vi "Close Panel With Fade Out.vi"(8 "error in":errorcluster, 11 "Philips Dialog in":refnum<class "Flex UI Dialog.lvclass">) -> (0 "error out":errorcluster, 3 "Philips Dialog out":refnum<class "Flex UI Dialog.lvclass">)   [LabVIEW 2014, in "Flex UI Dialog.lvclass"]
doc: "If the dialog front panel was initially closed, close it. Otherwise do nothing."
uses:
  Flex UI Dialog.lvclass
  Flex UI Dialog.lvclass/Flex UI Dialog.ctl
  Flex UI (Parent)/Flex UI.lvclass/Flex UI.ctl
  <vilib>/LAVA/UI Tools/Fading/_Fade(I32)__lava_lib_ui_tools.vi
  Flex UI (Parent)/Flex UI.lvclass
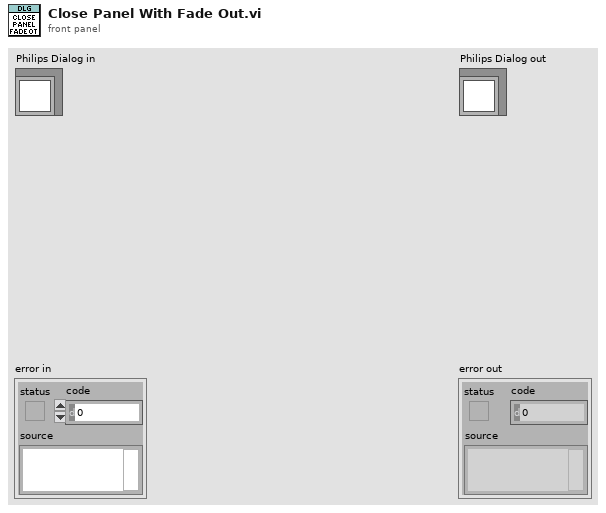
[diagram p1: front panel]
types:
  T1 = enum32{"invalid app kind", "Development System", "Run Time System", "Student Edition", "Embedded LabVIEW", "Evaluation", "Custom"}
  T2 = enum32{"Invalid", "Default", "Floating", "Floating/Auto-Hide", "Modal"}
  T3 = enum32{"Invalid", "Standard", "Closed", "Hidden", "Minimized", "Maximized"}
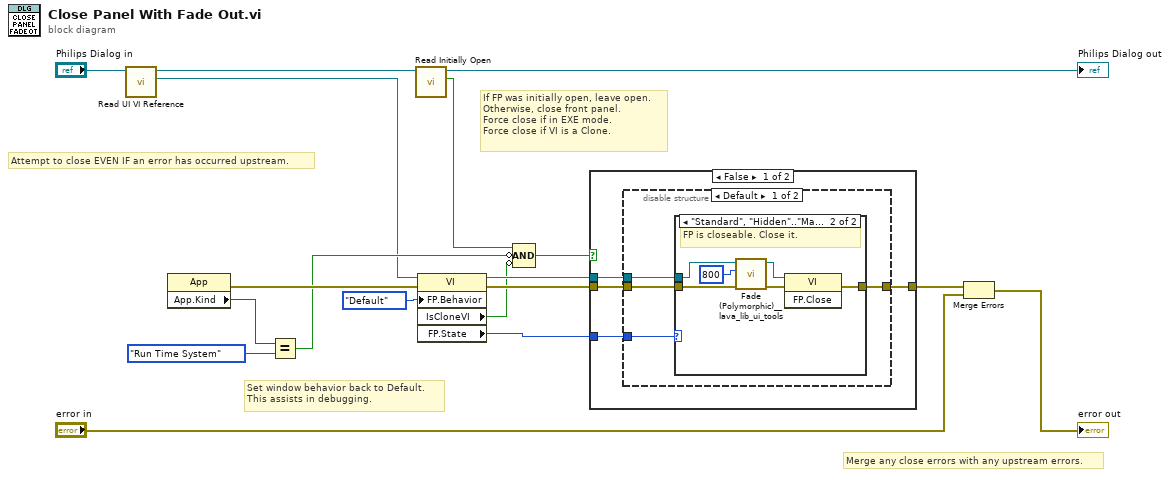
[diagram p0: block diagram]
diagram:
  # "Merge any close errors with any upstream errors."
  # "Attempt to close EVEN IF an error has occurred upstream."
  # "Set window behavior back to Default.\nThis assists in debugging."
  # "If FP was initially open, leave open.\nOtherwise, close front panel.\nForce close if in EXE mode.\nForce close if VI is a Clone."
  n1 = call "Read UI VI Reference.vi"("Philips UI in"="Philips Dialog in") -> ("UI VI Reference"=w6:refnum<vi>, "Philips UI out"=w7:refnum<class "Flex UI Dialog.lvclass">)  [unwired: 9 in]
  n2 = property class="App"() -> (error out=w13:errorcluster, "App.Kind"=w11:T1)  [unwired: 2 in, 1 out]
  n3 = Equal?(x=w11, y=T1."Run Time System" ("Application:Kind")) -> (x = y?=w9:bool)
  n4 = call "Read Initially Open.vi"("Philips Dialog in"=w7) -> ("Initially Open?"=w4:bool, "Philips Dialog out"=→"Philips Dialog out":refnum<class "Flex UI Dialog.lvclass">)  [unwired: 9 in]
  n5 = property class="VI"(reference=w6, error in=w13, "FP.Behavior"=T2."Default" ("Front Panel Window:Behavior")) -> (reference out=w14:refnum<vi>, error out=w16:errorcluster, "IsCloneVI"=w8:bool, "FP.State"=w1:T3)
  n6 = Compound Arithmetic op=AND(w4, invert w9, invert w8) -> (w10:bool)
  n7 = case shown="False" w10 {
    tunnel: w16 -> [w22 w35]
    tunnel: w14 -> [w21 _]
    tunnel: [w20 w35] -> w17
    tunnel: w1 -> [w19 _]
    frame False {
      n8 = disable-structure shown="Default" {
        disable-tunnel: w22 -> [w26 w34]
        disable-tunnel: w21 -> [w25 _]
        disable-tunnel: [w24 w34] -> w20
        disable-tunnel: w19 -> [w23 _]
        frame condition #0 (active) {
          n9 = case shown="\"Standard\", \"Hidden\"..\"Maximized\"" w23 {
            tunnel: w26 -> [w27 w32]
            tunnel: w25 -> [_ w30]
            tunnel: [w27 w33] -> w24
            frame "Invalid", Default {
              # "By default, do nothing."
            }
            frame "Standard", "Hidden".."Maximized" {
              # "FP is closeable. Close it."
              n10 = call-poly <vilib>:"Fade (Polymorphic)__lava_lib_ui_tools.vi"("error in"=w32, "Fade time (ms)"=800, "VI Reference (calling VI)"=w30) -> ("error out"=w31:errorcluster, "dup VI Reference"=w29:refnum<vi>)  [unwired: 7 in]
              n11 = invoke class="VI" method="FP.Close"(reference=w29, error in=w31) -> (error out=w33:errorcluster)  [unwired: 1 in, 2 out]
            }
          }
        }
        frame condition #1 {
        }
      }
    }
    frame True {
    }
  }
  n12 = Merge Errors(w17, "error in") -> (→"error out":errorcluster)
